vi "Actor Core.vi"(8 "error in":errorcluster, 11 "JogMotionView in":refnum<class "JogMotionView.lvclass">) -> (0 "error out":errorcluster, 3 "Actor out":refnum<class "Actor.lvclass">)   [LabVIEW 2020, in "JogMotionView.lvlib" / "JogMotionView.lvclass"]
doc: "(<B>Filename</B>: Actor Framework.lvlib:Actor.lvclass:Actor Core.vi)\n\nReceives messages to the actor, reacts to them, and initiates any error handling that may shut the actor down.\n\nDescendant classes may override this VI to append parallel tasks for the actor to complete while it handles messages. Overrides use the Call Parent Class Method node."
uses:
  JogMotionView.lvclass
  <vilib>/ActorFramework/Actor/Actor.lvclass
  Controls/Axis_Control.ctl
  <vilib>/gpm_packages/@cs/mva-dialogbox/source/IDialogBox/IDialogBox/IDialogBox.lvclass
  Controls/Controls.lvlib
panel:
  in  "Start Run":bool
  in  "Axis":T1 caption="轴号"
  in  "Deceleration(mm/Sec^2)":dbl caption="减速度(mm/Sec^2)"
  in  "Acceleration(mm/Sec^2)":dbl caption="加速度(mm/Sec^2)"
  in  "velocity(mm/Sec)":dbl caption="速度(mm/Sec)"
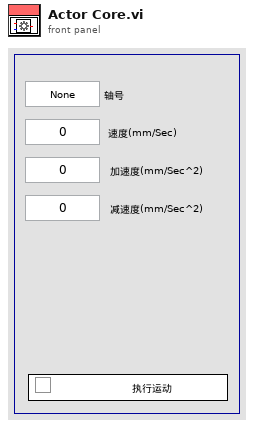
[diagram p1: front panel]
types:
  T1 = typedef "Controls.lvlib/Axis_Control.ctl" = enum16{"None", "1", "2", "3", "4", "5", "6", "7", "8"}
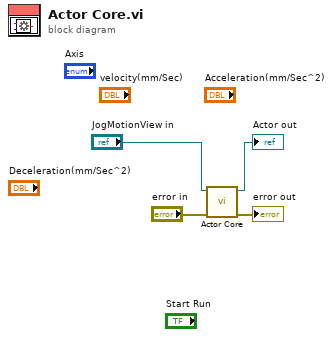
[diagram p0: block diagram]
diagram:
  n1 = call-parent "Actor Core.vi"("error in"="error in", "IViewable In"="JogMotionView in") -> ("error out"=→"error out":errorcluster, "Actor out"=→"Actor out":refnum<class "Actor.lvclass">)  [unwired: 8 in]
